vi "RTP_RTSP - Get SPS and PPS.vi"(7 "DESCRIBE":string) -> (8 "SPS":string, 10 "PPS":string)   [LabVIEW 2014]
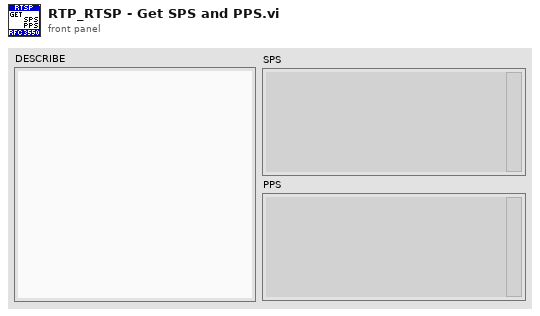
[diagram p1: front panel]
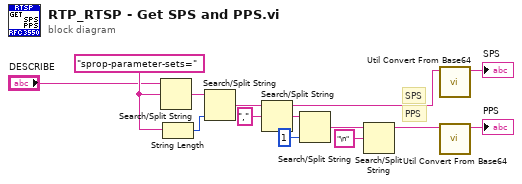
[diagram p0: block diagram]
diagram:
  w13 = "sprop-parameter-sets="
  # "PPS"
  # "SPS"
  n1 = Search/Split String(string="DESCRIBE", search string/char (-)=w13) -> (match + rest of string=w14:string)  [unwired: 1 in, 2 out]
  n2 = String Length(string=w13) -> (length=w12:i32)
  n3 = Search/Split String(string=w14, offset (0)=w12) -> (match + rest of string=w6:string)  [unwired: 1 in, 2 out]
  n4 = Search/Split String(string=w6, search string/char (-)=",") -> (substring before match=w8:string, match + rest of string=w7:string)  [unwired: 1 in, 1 out]
  n5 = Search/Split String(string=w7, offset (0)=1) -> (match + rest of string=w5:string)  [unwired: 1 in, 2 out]
  n6 = Search/Split String(string=w5, search string/char (-)="\n") -> (substring before match=w4:string)  [unwired: 1 in, 2 out]
  n7 = call "Util Convert From Base64.vi"("Base64 String"=w8) -> ("String"=→"SPS":string)  [unwired: 9 in, 1 out]
  n8 = call "Util Convert From Base64.vi"("Base64 String"=w4) -> ("String"=→"PPS":string)  [unwired: 9 in, 1 out]
